vi "Start Message Cycle.vi"(4 "Message Cycle Priority (Normal)":T2=enum."Normal", 5 "Last Message":refnum<class "Message.lvclass">, 6 "Cycle Timeout [ms] (-1)":i32=-1, 7 "Timeout Action":T1, 8 "error in (no error)":errorcluster, 9 "Inter-Message Wait [ms] (0)":i32, 10 "Message":refnum<class "Message.lvclass">, 11 "Message Enqueuer":refnum<class "Message Enqueuer.lvclass">) -> (0 "error out":errorcluster, 2 "Message Cycle Notifier":refnum<notifier>, 3 "Message Enqueuer out":refnum<class "Message Enqueuer.lvclass">)   [LabVIEW 2020, in "MessageCycle.lvclass"]
doc: "启动消息循环"
uses:
  MessageCycle.lvclass
  <vilib>/ActorFramework/Message Enqueuer/Message Enqueuer.lvclass
  <vilib>/ActorFramework/Message Enqueuer/Message Priority.ctl
  Message Cycle Notifications.ctl
  <vilib>/ActorFramework/Message/Message.lvclass
  C:/Program Files/National Instruments/LabVIEW 2020/vi.lib/ActorFramework/Message/Message.lvclass
  MessageCycle.lvclass/MessageCycle.ctl
  <vilib>/ActorFramework/Message Enqueuer/Message Enqueuer.lvclass/Message Enqueuer.ctl
  <vilib>/ActorFramework/Message Priority Queue/Priority Enqueue.vi
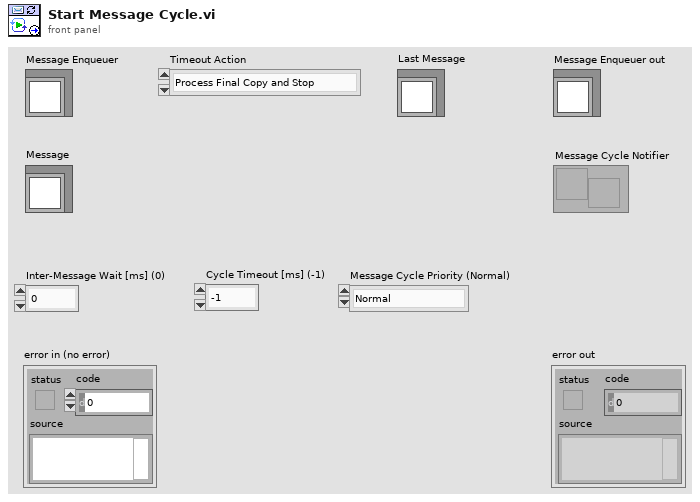
[diagram p1: front panel]
types:
  T1 = typedef "MessageCycle.lvclass/Message Cycle Notifications.ctl" = enum16{"Process Final Copy and Stop", "Stop Immediately", "Substitute Last Message and Stop"}
  T2 = typedef "Actor Framework.lvlib/Message Enqueuer.lvclass/Message Priority.ctl" = enum16{"Low", "Normal", "High"}
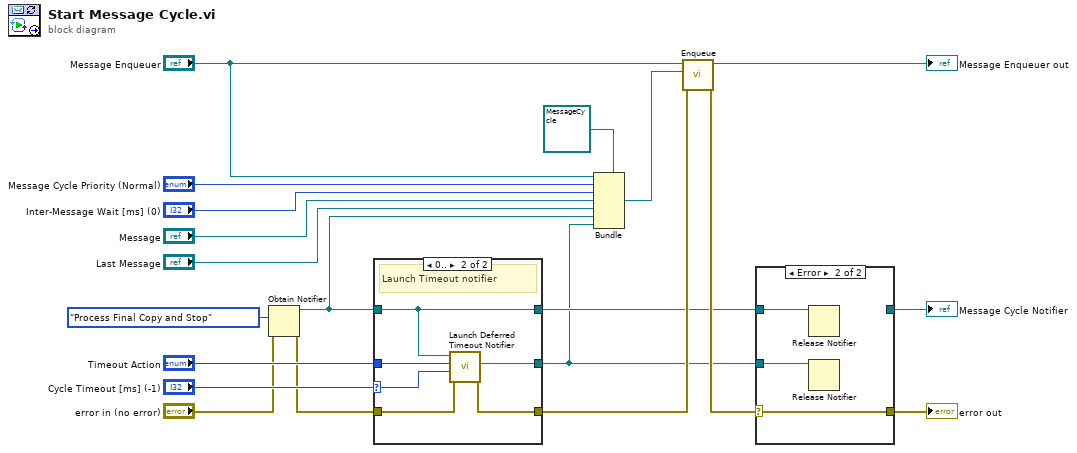
[diagram p0: block diagram]
diagram:
  n1 = Obtain Notifier(notification data type=Message_Cycle_Notifications."Process Final Copy and Stop", error in (no error)="error in (no error)") -> (notifier out=w4:refnum<notifier>, error out=w2:errorcluster)  [unwired: 2 in, 1 out]
  n2 = case shown="0.." "Cycle Timeout [ms] (-1)" {
    selector: "Cycle Timeout [ms] (-1)" -> [_ w24]
    tunnel: w2 -> [w22 w28]
    tunnel: [w22 w27] -> w11
    tunnel: w4 -> [w21 w25]
    tunnel: [_ w26] -> w1
    tunnel: [w21 w25] -> w9
    tunnel: "Timeout Action" -> [_ w23]
    frame ..-1 {
      # "No timeout"
    }
    frame 0.. {
      # "Launch Timeout notifier"
      n3 = call "Launch Deferred Timeout Notifier.vi"("error in (no error)"=w28, "Timeout [ms]"=w24, "Timeout Action"=w23, "Message Cycle Notifier"=w25) -> ("error out"=w27:errorcluster, "Timeout Notifier"=w26:refnum<notifier>)  [unwired: 6 in]
    }
  }
  n4 = Bundle(cluster=refnum<class "MessageCycle.lvclass"> refnum ("CyclicMessage in"), "Message Enqueuer", "Message Cycle Priority (Normal)", "Inter-Message Wait [ms] (0)", "Message", "Last Message", w4, w1) -> (w12:refnum<class "MessageCycle.lvclass">)
  n5 = call <vilib>:"Enqueue.vi"("error in (no error)"=w11, "Message"=w12, "Message Enqueuer in"="Message Enqueuer") -> ("error out"=w17:errorcluster, "Message Enqueuer out"=→"Message Enqueuer out":refnum<class "Message Enqueuer.lvclass">)  [unwired: 7 in]
  n6 = case shown="Error" w17 {
    selector: w17 -> [w29 w33]
    tunnel: w9 -> [w30 w32]
    tunnel: [w30 _] -> w6
    tunnel: [w29 w33] -> w16
    tunnel: w1 -> [_ w31]
    frame No Error {
    }
    frame Error {
      n7 = Release Notifier(notifier=w32) -> ()  [unwired: 2 in, 3 out]
      n8 = Release Notifier(notifier=w31) -> ()  [unwired: 2 in, 3 out]
    }
  }
  "error out" <- w16
  "Message Cycle Notifier" <- w6
